vi "Resolve Result Type.vi"(8 "error in (no error)":errorcluster, 10 "pStmt in":u64, 11 "#cols":i32) -> (0 "error out":errorcluster, 1 "Any blobs?":bool, 2 "blob?":bool[](array[boolean]), 3 "pStmt out":u64)   [LabVIEW 2020, in "sqlite3.lvlib"]
uses:
  sqlite3.lvlib
panel:
  out "Array - Numeric":i32[](array[numeric])
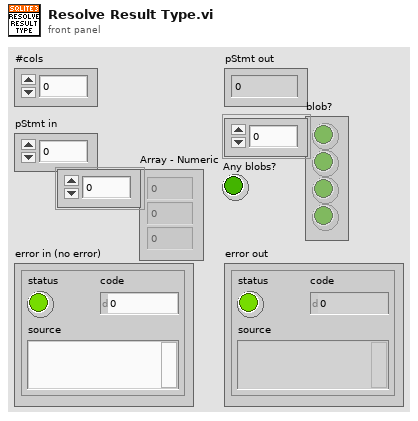
[diagram p1: front panel]
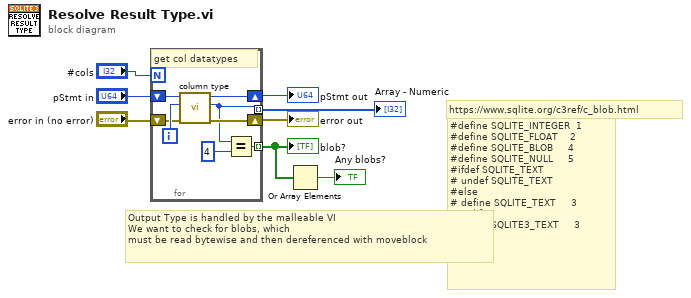
[diagram p0: block diagram]
diagram:
  # "Output Type is handled by the malleable VI\nWe want to check for blobs, which \nmust be read bytewise and then dereferenced with moveblock"
  # "https://www.sqlite.org/c3ref/c_blob.html"
  # "#define SQLITE_INTEGER  1\n#define SQLITE_FLOAT    2\n#define SQLITE_BLOB     4\n#define SQLITE_NULL     5\n#ifdef SQLITE_TEXT\n# undef SQLITE_TEXT\n#else\n# define SQLITE_TEXT     3\n#endif\n#define SQLITE3_TEXT     3"
  n1 = for {
    N: "#cols" -> [_]
    shift-right: [w14] -> w6
    shift-left: "error in (no error)" -> [w13]
    shift-right: [w12] -> w7
    shift-left: "pStmt in" -> [w16]
    tunnel: [w10] -> w3 mode=indexing
    tunnel: [w9] -> w1 mode=indexing
    i -> [w15]
    # "get col datatypes"
    n2 = call "column type.vi"("error in (no error)"=w13, "iCol"=w15, "para0"=w16) -> ("error out"=w14:errorcluster, "function return"=w9:i32, "para0 out"=w12:u64)  [unwired: 6 in]
    n3 = Equal?(x=w9, y=4) -> (x = y?=w10:bool)
  }
  "pStmt out" <- w7
  "error out" <- w6
  "blob?" <- w3
  "Array - Numeric" <- w1
  n4 = Or Array Elements(Boolean array=w3) -> (logical OR=→"Any blobs?":bool)
